vi "ImageToCustomPalette.vi"(4 "user maximum":dbl, 6 "user minimum":dbl, 7 "autoscale":bool=TRUE, 8 "error in (no error)":errorcluster, 9 "palette":T1(ring), 10 "dest image":T2, 11 "source image":T2) -> (0 "error out":errorcluster, 3 "output image":T2 caption="dest image")   [LabVIEW 2017]
uses:
  <vilib>/vision/Image Controls.llb/IMAQ Image.ctl
  <vilib>/vision/NI_Vision_Development_Module.lvlib
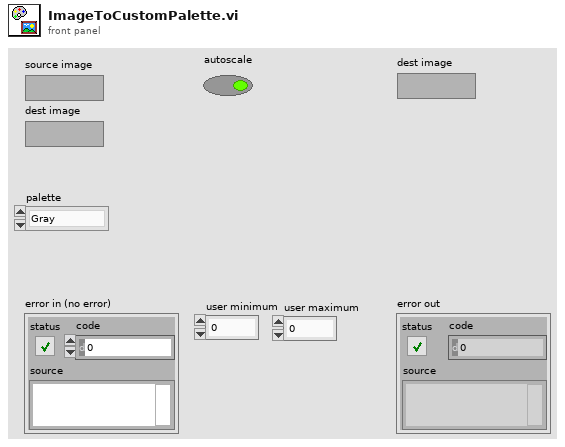
[diagram p1: front panel]
types:
  T1 = enum16{"Gray", "Binary", "Gradient", "Rainbow", "Temperature", "Full Rainbow", "Iron"}
  T2 = typedef "IMAQ Image.ctl" = refnum<image>
  T3 = enum32{"Gray", "Binary", "Gradient", "Rainbow", "Temperature"}
  T4 = cluster{"Numeric":u8, "Numeric 2":u8, "Numeric 3":u8}[]
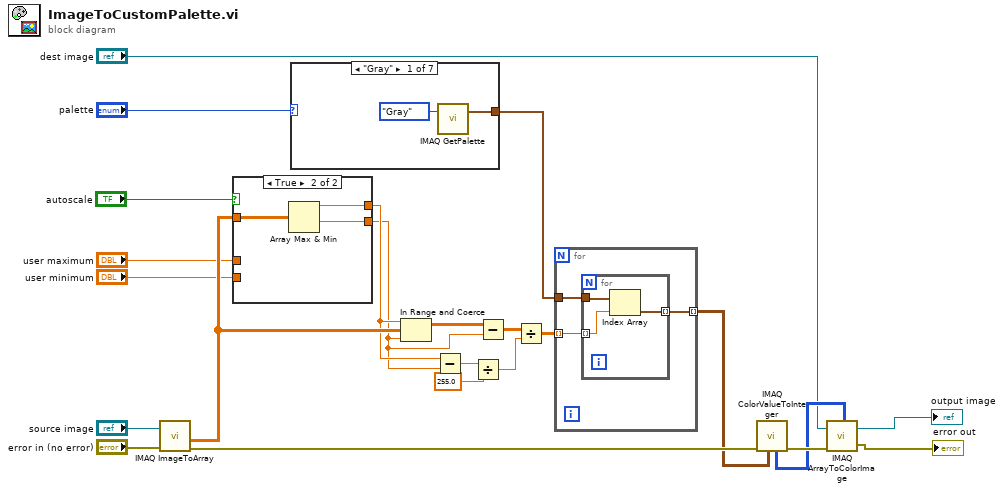
[diagram p0: block diagram]
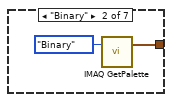
[diagram p2: hidden frame]
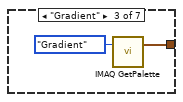
[diagram p3: hidden frame]
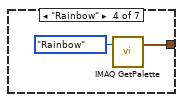
[diagram p4: hidden frame]
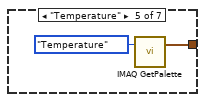
[diagram p5: hidden frame]
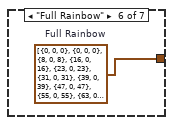
[diagram p6: hidden frame]
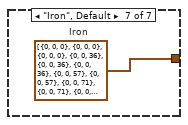
[diagram p7: hidden frame]
diagram:
  n1 = call "IMAQ ImageToArray"("error in (no error)"="error in (no error)", "Image"="source image") -> ("Image Pixels (Float)"=w6:sgl[][], "error out"=w14:errorcluster)  [unwired: 2 in, 3 out]
  n2 = case shown="True" "autoscale" {
    tunnel: w6 -> [_ w28]
    tunnel: [w25 w27] -> w5
    tunnel: [w24 w26] -> w4
    tunnel: "user maximum" -> [w25 _]
    tunnel: "user minimum" -> [w24 _]
    frame False {
    }
    frame True {
      n3 = Array Max & Min(array=w28) -> (max value=w27:sgl, min value=w26:sgl)  [unwired: 2 out]
    }
  }
  n4 = case shown="\"Gray\"" "palette" {
    tunnel: [w30 w32 w34 w36 w38 w39 w40] -> w15
    frame "Gray" {
      n5 = call "IMAQ GetPalette"("Palette Number (gray)"=T3."Gray") -> ("Color Palette"=w30:cluster{"Red":u8, "Green":u8, "Blue":u8}[])  [unwired: 4 in, 1 out]
    }
    frame "Binary" {
      n6 = call "IMAQ GetPalette"("Palette Number (gray)"=T3."Binary") -> ("Color Palette"=w32:cluster{"Red":u8, "Green":u8, "Blue":u8}[])  [unwired: 4 in, 1 out]
    }
    frame "Gradient" {
      n7 = call "IMAQ GetPalette"("Palette Number (gray)"=T3."Gradient") -> ("Color Palette"=w34:cluster{"Red":u8, "Green":u8, "Blue":u8}[])  [unwired: 4 in, 1 out]
    }
    frame "Rainbow" {
      n8 = call "IMAQ GetPalette"("Palette Number (gray)"=T3."Rainbow") -> ("Color Palette"=w36:cluster{"Red":u8, "Green":u8, "Blue":u8}[])  [unwired: 4 in, 1 out]
    }
    frame "Temperature" {
      n9 = call "IMAQ GetPalette"("Palette Number (gray)"=T3."Temperature") -> ("Color Palette"=w38:cluster{"Red":u8, "Green":u8, "Blue":u8}[])  [unwired: 4 in, 1 out]
    }
    frame "Full Rainbow" {
      w39 = T4 [{"Numeric"=0, "Numeric 2"=0, "Numeric 3"=0}, {"Numeric"=0, "Numeric 2"=0, "Numeric 3"=0}, {"Numeric"=8, "Numeric 2"=0, "Numeric 3"=8}, {"Numeric"=16, "Numeric 2"=0, "Numeric 3"=16}, {"Numeric"=23, "Numeric 2"=0, "Numeric 3"=23}, {"Numeric"=31, "Numeric 2"=0, "Numeric 3"=31}, {"Numeric"=39, "Numeric 2"=0, "Numeric 3"=39}, {"Numeric"=47, "Numeric 2"=0, "Numeric 3"=47}, {"Numeric"=55, "Numeric 2"=0, "Numeric 3"=55}, {"Numeric"=63, "Numeric 2"=0, "Numeric 3"=63}, {"Numeric"=71, "Numeric 2"=0, "Numeric 3"=71}, {"Numeric"=79, "Numeric 2"=0, "Numeric 3"=79}, {"Numeric"=84, "Numeric 2"=0, "Numeric 3"=84}, {"Numeric"=89, "Numeric 2"=0, "Numeric 3"=89}, {"Numeric"=94, "Numeric 2"=0, "Numeric 3"=94}, {"Numeric"=103, "Numeric 2"=0, "Numeric 3"=103}, {"Numeric"=111, "Numeric 2"=0, "Numeric 3"=111}, {"Numeric"=119, "Numeric 2"=0, "Numeric 3"=119}, {"Numeric"=127, "Numeric 2"=0, "Numeric 3"=127}, {"Numeric"=135, "Numeric 2"=0, "Numeric 3"=135}, {"Numeric"=143, "Numeric 2"=0, "Numeric 3"=143}, {"Numeric"=151, "Numeric 2"=0, "Numeric 3"=151}, {"Numeric"=159, "Numeric 2"=0, "Numeric 3"=159}, {"Numeric"=167, "Numeric 2"=0, "Numeric 3"=167}, {"Numeric"=175, "Numeric 2"=0, "Numeric 3"=175}, {"Numeric"=183, "Numeric 2"=0, "Numeric 3"=183}, {"Numeric"=191, "Numeric 2"=0, "Numeric 3"=191}, {"Numeric"=196, "Numeric 2"=0, "Numeric 3"=196}, {"Numeric"=201, "Numeric 2"=0, "Numeric 3"=201}, {"Numeric"=206, "Numeric 2"=0, "Numeric 3"=206}, {"Numeric"=215, "Numeric 2"=0, "Numeric 3"=215}, {"Numeric"=223, "Numeric 2"=0, "Numeric 3"=223}, {"Numeric"=231, "Numeric 2"=0, "Numeric 3"=231}, {"Numeric"=239, "Numeric 2"=0, "Numeric 3"=239}, {"Numeric"=247, "Numeric 2"=0, "Numeric 3"=247}, {"Numeric"=255, "Numeric 2"=0, "Numeric 3"=255}, {"Numeric"=247, "Numeric 2"=0, "Numeric 3"=253}, {"Numeric"=239, "Numeric 2"=0, "Numeric 3"=251}, {"Numeric"=231, "Numeric 2"=0, "Numeric 3"=248}, {"Numeric"=223, "Numeric 2"=0, "Numeric 3"=246}, {"Numeric"=218, "Numeric 2"=0, "Numeric 3"=243}, {"Numeric"=213, "Numeric 2"=0, "Numeric 3"=241}, {"Numeric"=208, "Numeric 2"=0, "Numeric 3"=239}, {"Numeric"=199, "Numeric 2"=0, "Numeric 3"=238}, {"Numeric"=191, "Numeric 2"=0, "Numeric 3"=236}, {"Numeric"=183, "Numeric 2"=0, "Numeric 3"=234}, {"Numeric"=175, "Numeric 2"=0, "Numeric 3"=232}, {"Numeric"=167, "Numeric 2"=0, "Numeric 3"=229}, {"Numeric"=159, "Numeric 2"=0, "Numeric 3"=227}, {"Numeric"=151, "Numeric 2"=0, "Numeric 3"=224}, {"Numeric"=143, "Numeric 2"=0, "Numeric 3"=222}, {"Numeric"=135, "Numeric 2"=0, "Numeric 3"=220}, {"Numeric"=127, "Numeric 2"=0, "Numeric 3"=218}, {"Numeric"=119, "Numeric 2"=0, "Numeric 3"=215}, {"Numeric"=111, "Numeric 2"=0, "Numeric 3"=213}, {"Numeric"=106, "Numeric 2"=0, "Numeric 3"=211}, {"Numeric"=101, "Numeric 2"=0, "Numeric 3"=210}, {"Numeric"=96, "Numeric 2"=0, "Numeric 3"=209}, {"Numeric"=87, "Numeric 2"=0, "Numeric 3"=206}, {"Numeric"=79, "Numeric 2"=0, "Numeric 3"=204}, {"Numeric"=71, "Numeric 2"=0, "Numeric 3"=201}, {"Numeric"=63, "Numeric 2"=0, "Numeric 3"=199}, {"Numeric"=55, "Numeric 2"=0, "Numeric 3"=196}, {"Numeric"=47, "Numeric 2"=0, "Numeric 3"=194}, {"Numeric"=39, "Numeric 2"=0, "Numeric 3"=192}, {"Numeric"=31, "Numeric 2"=0, "Numeric 3"=190}, {"Numeric"=23, "Numeric 2"=0, "Numeric 3"=187}, {"Numeric"=15, "Numeric 2"=0, "Numeric 3"=185}, {"Numeric"=7, "Numeric 2"=0, "Numeric 3"=182}, {"Numeric"=0, "Numeric 2"=0, "Numeric 3"=180}, {"Numeric"=0, "Numeric 2"=5, "Numeric 3"=181}, {"Numeric"=0, "Numeric 2"=10, "Numeric 3"=182}, {"Numeric"=0, "Numeric 2"=15, "Numeric 3"=183}, {"Numeric"=0, "Numeric 2"=31, "Numeric 3"=188}, {"Numeric"=0, "Numeric 2"=47, "Numeric 3"=193}, {"Numeric"=0, "Numeric 2"=55, "Numeric 3"=196}, {"Numeric"=0, "Numeric 2"=63, "Numeric 3"=198}, {"Numeric"=0, "Numeric 2"=71, "Numeric 3"=200}, {"Numeric"=0, "Numeric 2"=79, "Numeric 3"=202}, {"Numeric"=0, "Numeric 2"=87, "Numeric 3"=205}, {"Numeric"=0, "Numeric 2"=95, "Numeric 3"=207}, {"Numeric"=0, "Numeric 2"=100, "Numeric 3"=209}, {"Numeric"=0, "Numeric 2"=105, "Numeric 3"=210}, {"Numeric"=0, "Numeric 2"=110, "Numeric 3"=211}, {"Numeric"=0, "Numeric 2"=119, "Numeric 3"=214}, {"Numeric"=0, "Numeric 2"=127, "Numeric 3"=216}, {"Numeric"=0, "Numeric 2"=127, "Numeric 3"=216}, {"Numeric"=0, "Numeric 2"=135, "Numeric 3"=219}, {"Numeric"=0, "Numeric 2"=143, "Numeric 3"=221}, {"Numeric"=0, "Numeric 2"=151, "Numeric 3"=224}, {"Numeric"=0, "Numeric 2"=159, "Numeric 3"=226}, {"Numeric"=0, "Numeric 2"=167, "Numeric 3"=228}, {"Numeric"=0, "Numeric 2"=175, "Numeric 3"=230}, {"Numeric"=0, "Numeric 2"=191, "Numeric 3"=235}, {"Numeric"=0, "Numeric 2"=199, "Numeric 3"=238}, {"Numeric"=0, "Numeric 2"=207, "Numeric 3"=240}, {"Numeric"=0, "Numeric 2"=212, "Numeric 3"=242}, {"Numeric"=0, "Numeric 2"=217, "Numeric 3"=244}, {"Numeric"=0, "Numeric 2"=222, "Numeric 3"=246}, {"Numeric"=0, "Numeric 2"=231, "Numeric 3"=247}, {"Numeric"=0, "Numeric 2"=239, "Numeric 3"=249}, {"Numeric"=0, "Numeric 2"=247, "Numeric 3"=252}, {"Numeric"=0, "Numeric 2"=255, "Numeric 3"=254}, {"Numeric"=0, "Numeric 2"=250, "Numeric 3"=247}, {"Numeric"=0, "Numeric 2"=245, "Numeric 3"=239}, {"Numeric"=0, "Numeric 2"=241, "Numeric 3"=231}, {"Numeric"=0, "Numeric 2"=237, "Numeric 3"=223}, {"Numeric"=0, "Numeric 2"=232, "Numeric 3"=215}, {"Numeric"=0, "Numeric 2"=228, "Numeric 3"=207}, {"Numeric"=0, "Numeric 2"=224, "Numeric 3"=202}, {"Numeric"=0, "Numeric 2"=221, "Numeric 3"=197}, {"Numeric"=0, "Numeric 2"=218, "Numeric 3"=192}, {"Numeric"=0, "Numeric 2"=214, "Numeric 3"=183}, {"Numeric"=0, "Numeric 2"=210, "Numeric 3"=175}, {"Numeric"=0, "Numeric 2"=205, "Numeric 3"=167}, {"Numeric"=0, "Numeric 2"=201, "Numeric 3"=159}, {"Numeric"=0, "Numeric 2"=196, "Numeric 3"=151}, {"Numeric"=0, "Numeric 2"=192, "Numeric 3"=143}, {"Numeric"=0, "Numeric 2"=187, "Numeric 3"=135}, {"Numeric"=0, "Numeric 2"=183, "Numeric 3"=127}, {"Numeric"=0, "Numeric 2"=178, "Numeric 3"=119}, {"Numeric"=0, "Numeric 2"=174, "Numeric 3"=111}, {"Numeric"=0, "Numeric 2"=169, "Numeric 3"=103}, {"Numeric"=0, "Numeric 2"=165, "Numeric 3"=95}, {"Numeric"=0, "Numeric 2"=161, "Numeric 3"=90}, {"Numeric"=0, "Numeric 2"=158, "Numeric 3"=85}, {"Numeric"=0, "Numeric 2"=155, "Numeric 3"=80}, {"Numeric"=0, "Numeric 2"=151, "Numeric 3"=71}, {"Numeric"=0, "Numeric 2"=147, "Numeric 3"=63}, {"Numeric"=0, "Numeric 2"=142, "Numeric 3"=55}, {"Numeric"=0, "Numeric 2"=138, "Numeric 3"=47}, {"Numeric"=0, "Numeric 2"=133, "Numeric 3"=39}, {"Numeric"=0, "Numeric 2"=129, "Numeric 3"=31}, {"Numeric"=0, "Numeric 2"=124, "Numeric 3"=23}, {"Numeric"=0, "Numeric 2"=120, "Numeric 3"=15}, {"Numeric"=0, "Numeric 2"=115, "Numeric 3"=7}, {"Numeric"=0, "Numeric 2"=111, "Numeric 3"=0}, {"Numeric"=8, "Numeric 2"=114, "Numeric 3"=0}, {"Numeric"=16, "Numeric 2"=118, "Numeric 3"=0}, {"Numeric"=20, "Numeric 2"=121, "Numeric 3"=0}, {"Numeric"=25, "Numeric 2"=124, "Numeric 3"=0}, {"Numeric"=30, "Numeric 2"=127, "Numeric 3"=0}, {"Numeric"=38, "Numeric 2"=131, "Numeric 3"=0}, {"Numeric"=46, "Numeric 2"=135, "Numeric 3"=0}, {"Numeric"=53, "Numeric 2"=139, "Numeric 3"=0}, {"Numeric"=61, "Numeric 2"=143, "Numeric 3"=0}, {"Numeric"=68, "Numeric 2"=148, "Numeric 3"=0}, {"Numeric"=76, "Numeric 2"=152, "Numeric 3"=0}, {"Numeric"=83, "Numeric 2"=156, "Numeric 3"=0}, {"Numeric"=91, "Numeric 2"=160, "Numeric 3"=0}, {"Numeric"=98, "Numeric 2"=165, "Numeric 3"=0}, {"Numeric"=106, "Numeric 2"=169, "Numeric 3"=0}, {"Numeric"=106, "Numeric 2"=169, "Numeric 3"=0}, {"Numeric"=110, "Numeric 2"=172, "Numeric 3"=0}, {"Numeric"=115, "Numeric 2"=175, "Numeric 3"=0}, {"Numeric"=120, "Numeric 2"=178, "Numeric 3"=0}, {"Numeric"=128, "Numeric 2"=182, "Numeric 3"=0}, {"Numeric"=136, "Numeric 2"=186, "Numeric 3"=0}, {"Numeric"=143, "Numeric 2"=190, "Numeric 3"=0}, {"Numeric"=151, "Numeric 2"=194, "Numeric 3"=0}, {"Numeric"=158, "Numeric 2"=199, "Numeric 3"=0}, {"Numeric"=166, "Numeric 2"=203, "Numeric 3"=0}, {"Numeric"=173, "Numeric 2"=207, "Numeric 3"=0}, {"Numeric"=181, "Numeric 2"=211, "Numeric 3"=0}, {"Numeric"=188, "Numeric 2"=216, "Numeric 3"=0}, {"Numeric"=196, "Numeric 2"=220, "Numeric 3"=0}, {"Numeric"=203, "Numeric 2"=224, "Numeric 3"=0}, {"Numeric"=211, "Numeric 2"=228, "Numeric 3"=0}, {"Numeric"=215, "Numeric 2"=232, "Numeric 3"=0}, {"Numeric"=220, "Numeric 2"=235, "Numeric 3"=0}, {"Numeric"=233, "Numeric 2"=241, "Numeric 3"=0}, {"Numeric"=241, "Numeric 2"=245, "Numeric 3"=0}, {"Numeric"=248, "Numeric 2"=250, "Numeric 3"=0}, {"Numeric"=255, "Numeric 2"=254, "Numeric 3"=0}, {"Numeric"=253, "Numeric 2"=247, "Numeric 3"=0}, {"Numeric"=251, "Numeric 2"=239, "Numeric 3"=0}, {"Numeric"=249, "Numeric 2"=232, "Numeric 3"=0}, {"Numeric"=247, "Numeric 2"=224, "Numeric 3"=0}, {"Numeric"=246, "Numeric 2"=217, "Numeric 3"=0}, {"Numeric"=244, "Numeric 2"=209, "Numeric 3"=0}, {"Numeric"=244, "Numeric 2"=205, "Numeric 3"=0}, {"Numeric"=243, "Numeric 2"=200, "Numeric 3"=0}, {"Numeric"=242, "Numeric 2"=195, "Numeric 3"=0}, {"Numeric"=240, "Numeric 2"=187, "Numeric 3"=0}, {"Numeric"=238, "Numeric 2"=179, "Numeric 3"=0}, {"Numeric"=236, "Numeric 2"=172, "Numeric 3"=0}, {"Numeric"=234, "Numeric 2"=164, "Numeric 3"=0}, {"Numeric"=233, "Numeric 2"=157, "Numeric 3"=0}, {"Numeric"=231, "Numeric 2"=149, "Numeric 3"=0}, {"Numeric"=230, "Numeric 2"=142, "Numeric 3"=0}, {"Numeric"=228, "Numeric 2"=134, "Numeric 3"=0}, {"Numeric"=227, "Numeric 2"=127, "Numeric 3"=0}, {"Numeric"=225, "Numeric 2"=119, "Numeric 3"=0}, {"Numeric"=223, "Numeric 2"=112, "Numeric 3"=0}, {"Numeric"=221, "Numeric 2"=104, "Numeric 3"=0}, {"Numeric"=221, "Numeric 2"=100, "Numeric 3"=0}, {"Numeric"=220, "Numeric 2"=95, "Numeric 3"=0}, {"Numeric"=219, "Numeric 2"=90, "Numeric 3"=0}, {"Numeric"=217, "Numeric 2"=82, "Numeric 3"=0}, {"Numeric"=215, "Numeric 2"=74, "Numeric 3"=0}, {"Numeric"=214, "Numeric 2"=67, "Numeric 3"=0}, {"Numeric"=212, "Numeric 2"=59, "Numeric 3"=0}, {"Numeric"=210, "Numeric 2"=52, "Numeric 3"=0}, {"Numeric"=208, "Numeric 2"=44, "Numeric 3"=0}, {"Numeric"=207, "Numeric 2"=37, "Numeric 3"=0}, {"Numeric"=205, "Numeric 2"=29, "Numeric 3"=0}, {"Numeric"=204, "Numeric 2"=22, "Numeric 3"=0}, {"Numeric"=202, "Numeric 2"=14, "Numeric 3"=0}, {"Numeric"=201, "Numeric 2"=7, "Numeric 3"=0}, {"Numeric"=199, "Numeric 2"=0, "Numeric 3"=0}, {"Numeric"=201, "Numeric 2"=4, "Numeric 3"=4}, {"Numeric"=202, "Numeric 2"=8, "Numeric 3"=8}, {"Numeric"=203, "Numeric 2"=12, "Numeric 3"=12}, {"Numeric"=204, "Numeric 2"=17, "Numeric 3"=17}, {"Numeric"=206, "Numeric 2"=23, "Numeric 3"=23}, {"Numeric"=206, "Numeric 2"=29, "Numeric 3"=29}, {"Numeric"=207, "Numeric 2"=35, "Numeric 3"=35}, {"Numeric"=209, "Numeric 2"=40, "Numeric 3"=40}, {"Numeric"=211, "Numeric 2"=46, "Numeric 3"=46}, {"Numeric"=211, "Numeric 2"=52, "Numeric 3"=52}, {"Numeric"=212, "Numeric 2"=58, "Numeric 3"=58}, {"Numeric"=214, "Numeric 2"=63, "Numeric 3"=63}, {"Numeric"=216, "Numeric 2"=69, "Numeric 3"=69}, {"Numeric"=216, "Numeric 2"=73, "Numeric 3"=73}, {"Numeric"=217, "Numeric 2"=77, "Numeric 3"=77}, {"Numeric"=218, "Numeric 2"=81, "Numeric 3"=81}, {"Numeric"=219, "Numeric 2"=87, "Numeric 3"=87}, {"Numeric"=221, "Numeric 2"=93, "Numeric 3"=93}, {"Numeric"=221, "Numeric 2"=98, "Numeric 3"=98}, {"Numeric"=222, "Numeric 2"=104, "Numeric 3"=104}, {"Numeric"=224, "Numeric 2"=110, "Numeric 3"=110}, {"Numeric"=226, "Numeric 2"=116, "Numeric 3"=116}, {"Numeric"=226, "Numeric 2"=121, "Numeric 3"=121}, {"Numeric"=227, "Numeric 2"=127, "Numeric 3"=127}, {"Numeric"=229, "Numeric 2"=133, "Numeric 3"=133}, {"Numeric"=231, "Numeric 2"=139, "Numeric 3"=139}, {"Numeric"=231, "Numeric 2"=145, "Numeric 3"=145}, {"Numeric"=232, "Numeric 2"=151, "Numeric 3"=151}, {"Numeric"=233, "Numeric 2"=154, "Numeric 3"=154}, {"Numeric"=234, "Numeric 2"=158, "Numeric 3"=158}, {"Numeric"=235, "Numeric 2"=162, "Numeric 3"=162}, {"Numeric"=236, "Numeric 2"=168, "Numeric 3"=168}, {"Numeric"=237, "Numeric 2"=174, "Numeric 3"=174}, {"Numeric"=239, "Numeric 2"=179, "Numeric 3"=179}, {"Numeric"=241, "Numeric 2"=185, "Numeric 3"=185}, {"Numeric"=241, "Numeric 2"=191, "Numeric 3"=191}, {"Numeric"=242, "Numeric 2"=197, "Numeric 3"=197}, {"Numeric"=244, "Numeric 2"=203, "Numeric 3"=203}, {"Numeric"=246, "Numeric 2"=209, "Numeric 3"=209}, {"Numeric"=246, "Numeric 2"=214, "Numeric 3"=214}, {"Numeric"=247, "Numeric 2"=220, "Numeric 3"=220}, {"Numeric"=248, "Numeric 2"=224, "Numeric 3"=224}, {"Numeric"=249, "Numeric 2"=228, "Numeric 3"=228}, {"Numeric"=250, "Numeric 2"=232, "Numeric 3"=232}, {"Numeric"=253, "Numeric 2"=242, "Numeric 3"=242}, {"Numeric"=255, "Numeric 2"=255, "Numeric 3"=255}]  # Full Rainbow
    }
    frame "Iron", Default {
      w40 = cluster{"red":u8, "green":u8, "blue":u8}[] [{"red"=0, "green"=0, "blue"=0}, {"red"=0, "green"=0, "blue"=0}, {"red"=0, "green"=0, "blue"=0}, {"red"=0, "green"=0, "blue"=36}, {"red"=0, "green"=0, "blue"=36}, {"red"=0, "green"=0, "blue"=36}, {"red"=0, "green"=0, "blue"=57}, {"red"=0, "green"=0, "blue"=57}, {"red"=0, "green"=0, "blue"=71}, {"red"=0, "green"=0, "blue"=71}, {"red"=0, "green"=0, "blue"=71}, {"red"=2, "green"=0, "blue"=88}, {"red"=2, "green"=0, "blue"=88}, {"red"=4, "green"=0, "blue"=96}, {"red"=4, "green"=0, "blue"=96}, {"red"=4, "green"=0, "blue"=96}, {"red"=8, "green"=0, "blue"=107}, {"red"=8, "green"=0, "blue"=107}, {"red"=12, "green"=0, "blue"=117}, {"red"=12, "green"=0, "blue"=117}, {"red"=12, "green"=0, "blue"=117}, {"red"=17, "green"=0, "blue"=121}, {"red"=17, "green"=0, "blue"=121}, {"red"=17, "green"=0, "blue"=121}, {"red"=26, "green"=0, "blue"=128}, {"red"=26, "green"=0, "blue"=128}, {"red"=32, "green"=0, "blue"=132}, {"red"=32, "green"=0, "blue"=132}, {"red"=32, "green"=0, "blue"=132}, {"red"=42, "green"=0, "blue"=138}, {"red"=42, "green"=0, "blue"=138}, {"red"=49, "green"=0, "blue"=141}, {"red"=49, "green"=0, "blue"=141}, {"red"=49, "green"=0, "blue"=141}, {"red"=58, "green"=0, "blue"=145}, {"red"=58, "green"=0, "blue"=145}, {"red"=66, "green"=0, "blue"=149}, {"red"=66, "green"=0, "blue"=149}, {"red"=66, "green"=0, "blue"=149}, {"red"=71, "green"=0, "blue"=150}, {"red"=71, "green"=0, "blue"=150}, {"red"=80, "green"=0, "blue"=152}, {"red"=80, "green"=0, "blue"=152}, {"red"=80, "green"=0, "blue"=152}, {"red"=86, "green"=0, "blue"=153}, {"red"=86, "green"=0, "blue"=153}, {"red"=86, "green"=0, "blue"=153}, {"red"=95, "green"=0, "blue"=155}, {"red"=95, "green"=0, "blue"=155}, {"red"=101, "green"=0, "blue"=155}, {"red"=101, "green"=0, "blue"=155}, {"red"=101, "green"=0, "blue"=155}, {"red"=110, "green"=0, "blue"=156}, {"red"=110, "green"=0, "blue"=156}, {"red"=118, "green"=0, "blue"=157}, {"red"=118, "green"=0, "blue"=157}, {"red"=118, "green"=0, "blue"=157}, {"red"=124, "green"=0, "blue"=157}, {"red"=124, "green"=0, "blue"=157}, {"red"=132, "green"=0, "blue"=157}, {"red"=132, "green"=0, "blue"=157}, {"red"=132, "green"=0, "blue"=157}, {"red"=138, "green"=0, "blue"=157}, {"red"=138, "green"=0, "blue"=157}, {"red"=146, "green"=0, "blue"=156}, {"red"=146, "green"=0, "blue"=156}, {"red"=146, "green"=0, "blue"=156}, {"red"=152, "green"=0, "blue"=155}, {"red"=152, "green"=0, "blue"=155}, {"red"=152, "green"=0, "blue"=155}, {"red"=160, "green"=0, "blue"=155}, {"red"=160, "green"=0, "blue"=155}, {"red"=166, "green"=0, "blue"=154}, {"red"=166, "green"=0, "blue"=154}, {"red"=166, "green"=0, "blue"=154}, {"red"=170, "green"=0, "blue"=153}, {"red"=170, "green"=0, "blue"=153}, {"red"=176, "green"=1, "blue"=152}, {"red"=176, "green"=1, "blue"=152}, {"red"=176, "green"=1, "blue"=152}, {"red"=179, "green"=2, "blue"=151}, {"red"=179, "green"=2, "blue"=151}, {"red"=184, "green"=3, "blue"=149}, {"red"=184, "green"=3, "blue"=149}, {"red"=184, "green"=3, "blue"=149}, {"red"=188, "green"=5, "blue"=147}, {"red"=188, "green"=5, "blue"=147}, {"red"=188, "green"=5, "blue"=147}, {"red"=191, "green"=6, "blue"=146}, {"red"=191, "green"=6, "blue"=146}, {"red"=194, "green"=9, "blue"=144}, {"red"=194, "green"=9, "blue"=144}, {"red"=194, "green"=9, "blue"=144}, {"red"=196, "green"=12, "blue"=141}, {"red"=196, "green"=12, "blue"=141}, {"red"=200, "green"=16, "blue"=136}, {"red"=200, "green"=16, "blue"=136}, {"red"=200, "green"=16, "blue"=136}, {"red"=202, "green"=18, "blue"=133}, {"red"=202, "green"=18, "blue"=133}, {"red"=206, "green"=23, "blue"=127}, {"red"=206, "green"=23, "blue"=127}, {"red"=206, "green"=23, "blue"=127}, {"red"=209, "green"=27, "blue"=119}, {"red"=209, "green"=27, "blue"=119}, {"red"=211, "green"=30, "blue"=114}, {"red"=211, "green"=30, "blue"=114}, {"red"=211, "green"=30, "blue"=114}, {"red"=214, "green"=36, "blue"=106}, {"red"=214, "green"=36, "blue"=106}, {"red"=214, "green"=36, "blue"=106}, {"red"=217, "green"=40, "blue"=99}, {"red"=217, "green"=40, "blue"=99}, {"red"=219, "green"=46, "blue"=89}, {"red"=219, "green"=46, "blue"=89}, {"red"=219, "green"=46, "blue"=89}, {"red"=221, "green"=49, "blue"=79}, {"red"=221, "green"=49, "blue"=79}, {"red"=223, "green"=55, "blue"=62}, {"red"=223, "green"=55, "blue"=62}, {"red"=223, "green"=55, "blue"=62}, {"red"=226, "green"=60, "blue"=45}, {"red"=226, "green"=60, "blue"=45}, {"red"=228, "green"=63, "blue"=34}, {"red"=228, "green"=63, "blue"=34}, {"red"=228, "green"=63, "blue"=34}, {"red"=230, "green"=69, "blue"=24}, {"red"=230, "green"=69, "blue"=24}, {"red"=231, "green"=72, "blue"=20}, {"red"=231, "green"=72, "blue"=20}, {"red"=231, "green"=72, "blue"=20}, {"red"=233, "green"=77, "blue"=14}, {"red"=233, "green"=77, "blue"=14}, {"red"=233, "green"=77, "blue"=14}, {"red"=235, "green"=80, "blue"=11}, {"red"=235, "green"=80, "blue"=11}, {"red"=236, "green"=86, "blue"=8}, {"red"=236, "green"=86, "blue"=8}, {"red"=236, "green"=86, "blue"=8}, {"red"=237, "green"=91, "blue"=6}, {"red"=237, "green"=91, "blue"=6}, {"red"=238, "green"=94, "blue"=5}, {"red"=238, "green"=94, "blue"=5}, {"red"=238, "green"=94, "blue"=5}, {"red"=240, "green"=99, "blue"=4}, {"red"=240, "green"=99, "blue"=4}, {"red"=241, "green"=102, "blue"=3}, {"red"=241, "green"=102, "blue"=3}, {"red"=241, "green"=102, "blue"=3}, {"red"=241, "green"=106, "blue"=2}, {"red"=241, "green"=106, "blue"=2}, {"red"=241, "green"=106, "blue"=2}, {"red"=242, "green"=109, "blue"=1}, {"red"=242, "green"=109, "blue"=1}, {"red"=244, "green"=114, "blue"=1}, {"red"=244, "green"=114, "blue"=1}, {"red"=244, "green"=114, "blue"=1}, {"red"=244, "green"=119, "blue"=0}, {"red"=244, "green"=119, "blue"=0}, {"red"=245, "green"=123, "blue"=0}, {"red"=245, "green"=123, "blue"=0}, {"red"=245, "green"=123, "blue"=0}, {"red"=246, "green"=129, "blue"=0}, {"red"=246, "green"=129, "blue"=0}, {"red"=247, "green"=133, "blue"=0}, {"red"=247, "green"=133, "blue"=0}, {"red"=247, "green"=133, "blue"=0}, {"red"=248, "green"=137, "blue"=0}, {"red"=248, "green"=137, "blue"=0}, {"red"=249, "green"=142, "blue"=0}, {"red"=249, "green"=142, "blue"=0}, {"red"=249, "green"=142, "blue"=0}, {"red"=249, "green"=145, "blue"=0}, {"red"=249, "green"=145, "blue"=0}, {"red"=249, "green"=145, "blue"=0}, {"red"=250, "green"=150, "blue"=0}, {"red"=250, "green"=150, "blue"=0}, {"red"=251, "green"=154, "blue"=0}, {"red"=251, "green"=154, "blue"=0}, {"red"=251, "green"=154, "blue"=0}, {"red"=252, "green"=161, "blue"=0}, {"red"=252, "green"=161, "blue"=0}, {"red"=253, "green"=166, "blue"=0}, {"red"=253, "green"=166, "blue"=0}, {"red"=253, "green"=166, "blue"=0}, {"red"=253, "green"=171, "blue"=0}, {"red"=253, "green"=171, "blue"=0}, {"red"=254, "green"=177, "blue"=0}, {"red"=254, "green"=177, "blue"=0}, {"red"=254, "green"=177, "blue"=0}, {"red"=254, "green"=180, "blue"=0}, {"red"=254, "green"=180, "blue"=0}, {"red"=254, "green"=185, "blue"=0}, {"red"=254, "green"=185, "blue"=0}, {"red"=254, "green"=185, "blue"=0}, {"red"=254, "green"=189, "blue"=0}, {"red"=254, "green"=189, "blue"=0}, {"red"=254, "green"=189, "blue"=0}, {"red"=254, "green"=195, "blue"=0}, {"red"=254, "green"=195, "blue"=0}, {"red"=254, "green"=199, "blue"=0}, {"red"=254, "green"=199, "blue"=0}, {"red"=254, "green"=199, "blue"=0}, {"red"=254, "green"=203, "blue"=2}, {"red"=254, "green"=203, "blue"=2}, {"red"=254, "green"=208, "blue"=4}, {"red"=254, "green"=208, "blue"=4}, {"red"=254, "green"=208, "blue"=4}, {"red"=254, "green"=211, "blue"=7}, {"red"=254, "green"=211, "blue"=7}, {"red"=254, "green"=216, "blue"=12}, {"red"=254, "green"=216, "blue"=12}, {"red"=254, "green"=216, "blue"=12}, {"red"=255, "green"=219, "blue"=15}, {"red"=255, "green"=219, "blue"=15}, {"red"=255, "green"=219, "blue"=15}, {"red"=255, "green"=222, "blue"=26}, {"red"=255, "green"=222, "blue"=26}, {"red"=255, "green"=225, "blue"=34}, {"red"=255, "green"=225, "blue"=34}, {"red"=255, "green"=225, "blue"=34}, {"red"=255, "green"=229, "blue"=45}, {"red"=255, "green"=229, "blue"=45}, {"red"=255, "green"=232, "blue"=63}, {"red"=255, "green"=232, "blue"=63}, {"red"=255, "green"=232, "blue"=63}, {"red"=255, "green"=235, "blue"=75}, {"red"=255, "green"=235, "blue"=75}, {"red"=255, "green"=238, "blue"=93}, {"red"=255, "green"=238, "blue"=93}, {"red"=255, "green"=238, "blue"=93}, {"red"=255, "green"=240, "blue"=106}, {"red"=255, "green"=240, "blue"=106}, {"red"=255, "green"=242, "blue"=130}, {"red"=255, "green"=242, "blue"=130}, {"red"=255, "green"=242, "blue"=130}, {"red"=255, "green"=244, "blue"=144}, {"red"=255, "green"=244, "blue"=144}, {"red"=255, "green"=244, "blue"=144}, {"red"=255, "green"=246, "blue"=165}, {"red"=255, "green"=246, "blue"=165}, {"red"=255, "green"=248, "blue"=186}, {"red"=255, "green"=248, "blue"=186}, {"red"=255, "green"=248, "blue"=186}, {"red"=255, "green"=249, "blue"=197}, {"red"=255, "green"=249, "blue"=197}, {"red"=255, "green"=251, "blue"=214}, {"red"=255, "green"=251, "blue"=214}, {"red"=255, "green"=251, "blue"=214}, {"red"=255, "green"=253, "blue"=225}, {"red"=255, "green"=253, "blue"=225}, {"red"=255, "green"=255, "blue"=241}, {"red"=255, "green"=255, "blue"=241}, {"red"=255, "green"=255, "blue"=241}, {"red"=255, "green"=255, "blue"=255}, {"red"=255, "green"=255, "blue"=255}]  # Iron
    }
  }
  n10 = In Range and Coerce(upper limit=w5, x=w6, lower limit=w4) -> (coerced(x)=w20:dbl[][])  [unwired: 1 out]
  n11 = Subtract(x=w5, y=w4) -> (x-y=w19:dbl)
  n12 = Divide(x=w19, y=255.0) -> (x/y=w17:dbl)
  n13 = Subtract(x=w20, y=w4) -> (x-y=w21:dbl[][])
  n14 = Divide(x=w21, y=w17) -> (x/y=w16:dbl[][])
  n15 = for {
    tunnel: w16 -> [w43] mode=indexing
    tunnel: w15 -> [w42]
    tunnel: [w41] -> w13 mode=indexing
    n16 = for {
      tunnel: w43 -> [w45] mode=indexing
      tunnel: w42 -> [w46]
      tunnel: [w44] -> w41 mode=indexing
      n17 = Index Array(array=w46, index=w45) -> (element=w44:cluster{"red":u8, "green":u8, "blue":u8})
    }
  }
  n18 = call "IMAQ ColorValueToInteger"("error in (no error)"=w14, "2D Color value array"=w13) -> ("2D U32 array"=w11:u32[][], "error out"=w12:errorcluster)  [unwired: 3 in, 2 out]
  n19 = call "IMAQ ArrayToColorImage"("Image Pixels (U32)"=w11, "Image"="dest image", "error in (no error)"=w12) -> ("Image Out"=→"output image":T2, "error out"=→"error out":errorcluster)  [unwired: 2 in]
